vi "Phase359.vi"(11 "DataIn":waveform(dbl)) -> (3 "DataOut":waveform(dbl))   [LabVIEW 2018]
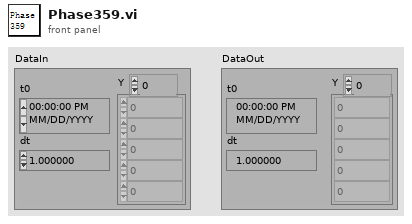
[diagram p1: front panel]
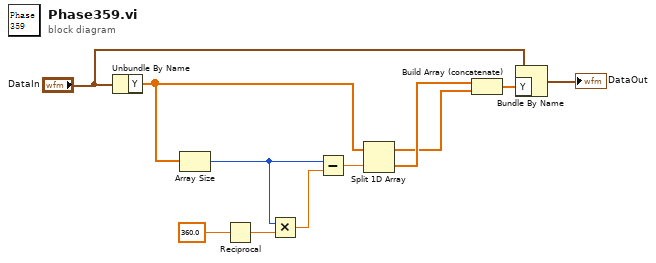
[diagram p0: block diagram]
diagram:
  n1 = Unbundle By Name("DataIn") -> ("Y"=w11:dbl[])
  n2 = Array Size(array=w11) -> (size(s)=w3:i32)
  n3 = Reciprocal(x=360.0) -> (1/x=w2:dbl)
  n4 = Multiply(x=w3, y=w2) -> (x*y=w1:dbl)
  n5 = Subtract(x=w3, y=w1) -> (x-y=w10:dbl)
  n6 = Split 1D Array(array=w11, index=w10) -> (first subarray=w8:dbl[], second subarray=w9:dbl[])
  n7 = Build Array (concatenate)(w9, w8) -> (w7:dbl[])
  n8 = Bundle By Name(cluster="DataIn", "Y"=w7) -> (→"DataOut":waveform(dbl))
